vi "Read Return Message Msg.vi"(8 "error in (no error)":errorcluster, 11 "Network Stream in":refnum<class "Network Stream.lvclass">) -> (0 "error out":errorcluster, 2 "Network Stream.lvlib:Network Stream Return Message Msg.lvclass":refnum<class "Return undeliverable Msg.lvclass">, 3 "Network Stream out":refnum<class "Network Stream.lvclass">)   [LabVIEW 2014]
uses:
  Network Stream.lvclass
  Proxy/Proxy Messages/Return undeliverable Msg/Return undeliverable Msg.lvclass
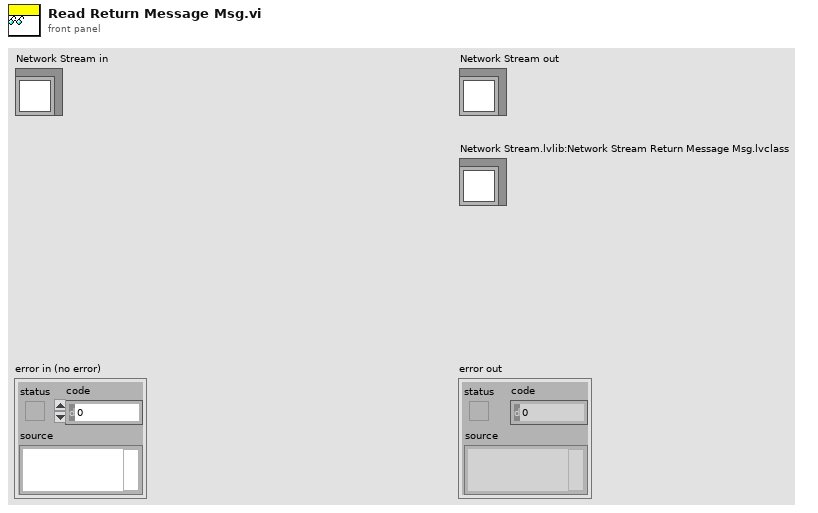
[diagram p1: front panel]
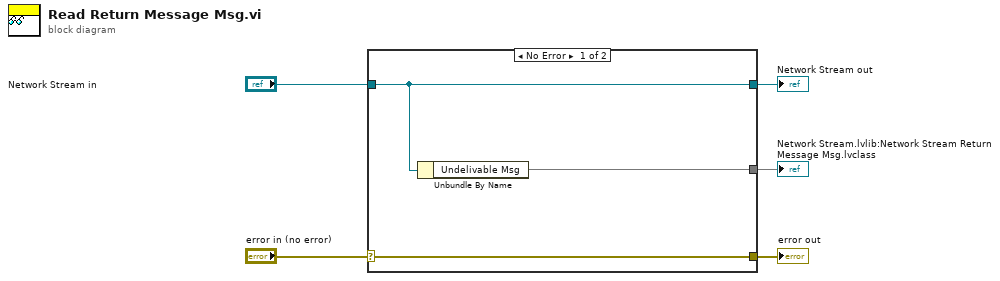
[diagram p0: block diagram]
diagram:
  n1 = case shown="No Error" "error in (no error)" {
    selector: "error in (no error)" -> [w8 w9]
    tunnel: [w8 w9] -> w4
    tunnel: [w7 w10] -> w2
    tunnel: "Network Stream in" -> [w7 w10]
    tunnel: [w6 _] -> w1
    frame No Error {
      n2 = Unbundle By Name(w7) -> ("Undelivable Msg"=w6)
    }
    frame Error {
    }
  }
  "error out" <- w4
  "Network Stream out" <- w2
  "Network Stream.lvlib:Network Stream Return Message Msg.lvclass" <- w1
